vi "Call NIPKG CLI.vi"(8 "error in (no error)":errorcluster, 11 "command":string) -> (0 "error out":errorcluster, 3 "command line standard output":string)   [LabVIEW 2014, in "NIPM_API.lvlib"]
doc: "This VI calls the nipkg.exe command-line interface (CLI) from the command line."
uses:
  NIPM_API.lvlib
  <vilib>/Utility/sysdir.llb/System Directory Type.ctl
panel:
  out "standard error":string
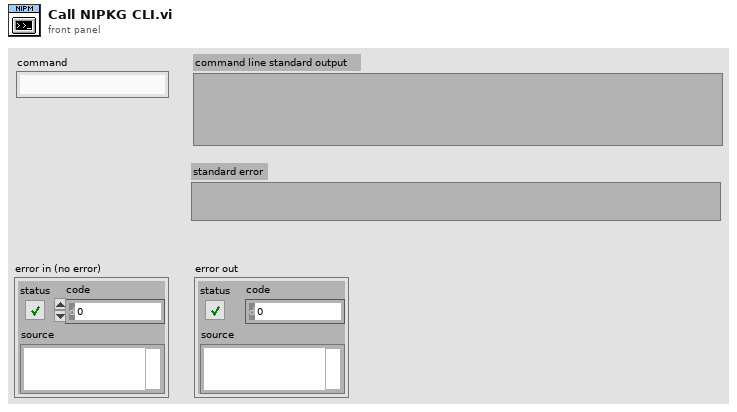
[diagram p1: front panel]
types:
  T1 = typedef "System Directory Type.ctl" = i32
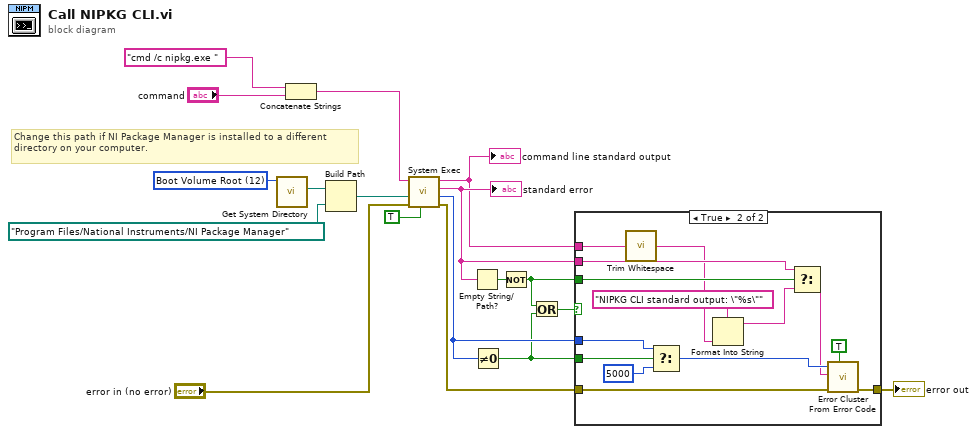
[diagram p0: block diagram]
diagram:
  w11 = T1 12 items=["User Home"=0, "User Desktop"=1, "User Documents"=2, "User Application Data"=3, "User Preferences"=4, "User Temporary"=5, "Public Documents"=6, "Public Application Data"=7, "Public Preferences"=8, "Public Cache"=13, "System Core Libraries"=9, "System Installed Libraries"=10, "Application Files"=11, "Boot Volume Root"=12] ("system directory type")
  # "Change this path if NI Package Manager is installed to a different directory on your computer."
  n1 = call <vilib>:"Get System Directory.vi"("system directory type"=w11) -> ("system directory"=w12:path)  [unwired: 10 in]
  n2 = Concatenate Strings("cmd /c nipkg.exe " ("string"), "command") -> (w8:string)
  n3 = Build Path(base path=w12, name or relative path=path "Program Files/National Instruments/NI Package Manager" ("working directory")) -> (appended path=w14:path)
  n4 = call <vilib>:"System Exec.vi"("run minimized? (F)"=TRUE, "error in (no error)"="error in (no error)", "working directory"=w14, "command line"=w8) -> ("error out"=w16:errorcluster, "return code"=w4:i32, "standard error"=w15:string, "standard output"=w1:string)  [unwired: 4 in]
  "command line standard output" <- w1
  "standard error" <- w15
  n5 = Empty String/Path?(string/path=w15) -> (empty?=w6:bool)
  n6 = Not Equal To 0?(x=w4) -> (x != 0?=w2:bool)
  n7 = Not(x=w6) -> (.not. x?=w3:bool)
  n8 = Or(x=w3, y=w2) -> (x .or. y?=w5:bool)
  n9 = case shown="True" w5 {
    tunnel: w16 -> [w19 w33]
    tunnel: w15 -> [_ w25]
    tunnel: [w19 w32] -> w17
    tunnel: w4 -> [_ w27]
    tunnel: w2 -> [_ w28]
    tunnel: w3 -> [_ w24]
    tunnel: w1 -> [_ w23]
    frame False {
    }
    frame True {
      n10 = call <vilib>:"Trim Whitespace.vi"("string"=w23) -> ("trimmed string"=w20:string)  [unwired: 1 in]
      n11 = Select(t=w27, s=w28, f=5000 ("error code (0)")) -> (s? t:f=w31:i32)
      n12 = Format Into String(format string="NIPKG CLI standard output: \"%s\"", w20) -> (resulting string=w21:string)  [unwired: 2 in, 1 out]
      n13 = Select(t=w25, s=w24, f=w21) -> (s? t:f=w29:string)
      n14 = call <vilib>:"Error Cluster From Error Code.vi"("show call chain? (False)"=TRUE, "error in (no error)"=w33, "error message (\"\")"=w29, "error code (0)"=w31) -> ("error out"=w32:errorcluster)  [unwired: 5 in]
    }
  }
  "error out" <- w17
